vi "Configure SPI Normal.vi"(6 "SPI Width (8)":dbl=8.0, 8 "error in (no error)":errorcluster, 9 "Bit Order (0: Least First)":i32(ring) items=["Least First", "Most First"], 10 "Channel (1: Serial Bus 1)":i32(ring)=1 items=["Serial Bus 1"=1, "Serial Bus 2"=2, "Serial Bus 3"=3, "Serial Bus 4"=4], 11 "VISA resource name":refnum<visa-resource-name>) -> (0 "error out":errorcluster, 3 "VISA resource name out":refnum<visa-resource-name>)   [LabVIEW 2020, in "Agilent 90000 Series.lvlib"]
doc: "Configures general settings of SPI serial bus."
uses:
  Agilent 90000 Series.lvlib
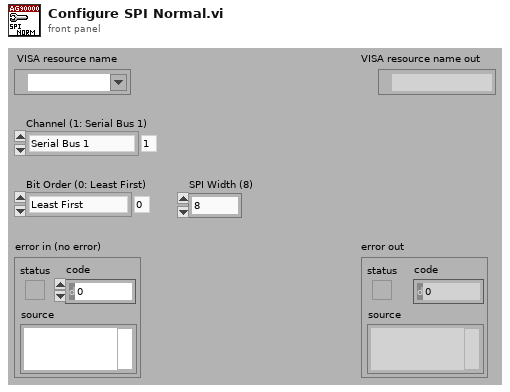
[diagram p1: front panel]
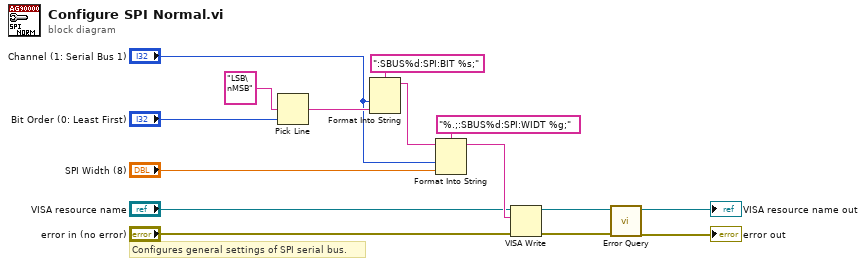
[diagram p0: block diagram]
diagram:
  # "Configures general settings of SPI serial bus."
  n1 = Pick Line(multi-line string="LSB\nMSB", line index="Bit Order (0: Least First)") -> (output string=w12:string)  [unwired: 1 out]
  n2 = Format Into String(format string=":SBUS%d:SPI:BIT %s;", "Channel (1: Serial Bus 1)", w12) -> (resulting string=w2:string)  [unwired: 2 in, 1 out]
  n3 = Format Into String(format string="%.;:SBUS%d:SPI:WIDT %g;", initial string=w2, "Channel (1: Serial Bus 1)", "SPI Width (8)") -> (resulting string=w9:string)  [unwired: 1 in, 1 out]
  n4 = VISA Write(VISA resource name="VISA resource name", write buffer=w9, error in (no error)="error in (no error)") -> (VISA resource name out=w6:refnum<visa-resource-name>, error out=w5:errorcluster)  [unwired: 1 out]
  n5 = call "Error Query.vi"("error in (no error)"=w5, "VISA resource name"=w6) -> ("error out"=→"error out":errorcluster, "VISA resource name out"=→"VISA resource name out":refnum<visa-resource-name>)  [unwired: 8 out]
